vi "test Undeployment Returns to Default State.vi"(8 "error in (no error)":errorcluster, 11 "TestCase in":refnum<class "NI-SWITCH System Tests.lvclass">) -> (0 "error out":errorcluster, 3 "TestCase out":refnum<class "NI-SWITCH System Tests.lvclass">)   [LabVIEW 2017, in "NI-SWITCH System Tests.lvclass"]
uses:
  NI-SWITCH System Tests.lvclass
  SLSC Switch States.ctl
  NI-SWITCH System Tests.lvclass/NI-SWITCH System Tests.ctl
  <vilib>/addons/_JKI Toolkits/VI Tester/TestCase.llb/TestCase.lvclass
  C:/Program Files (x86)/National Instruments/LabVIEW 2017/vi.lib/addons/_JKI Toolkits/VI Tester/TestCase.llb/TestCase.lvclass
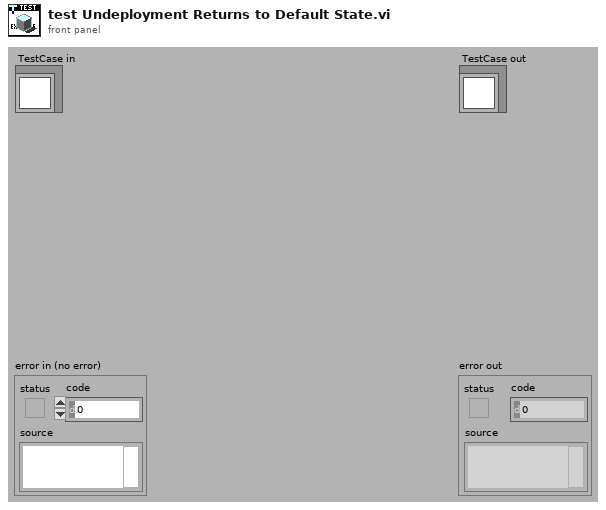
[diagram p1: front panel]
types:
  T1 = typedef "NI-SWITCH System Tests.lvclass/SLSC Switch States.ctl" = cluster{"Channel Load States":cluster{"name":string, "value":i32}[], "Channel Bus States":cluster{"name":string, "value":i32}[], "Channel Pair States":cluster{"name":string, "value":i32}[]}
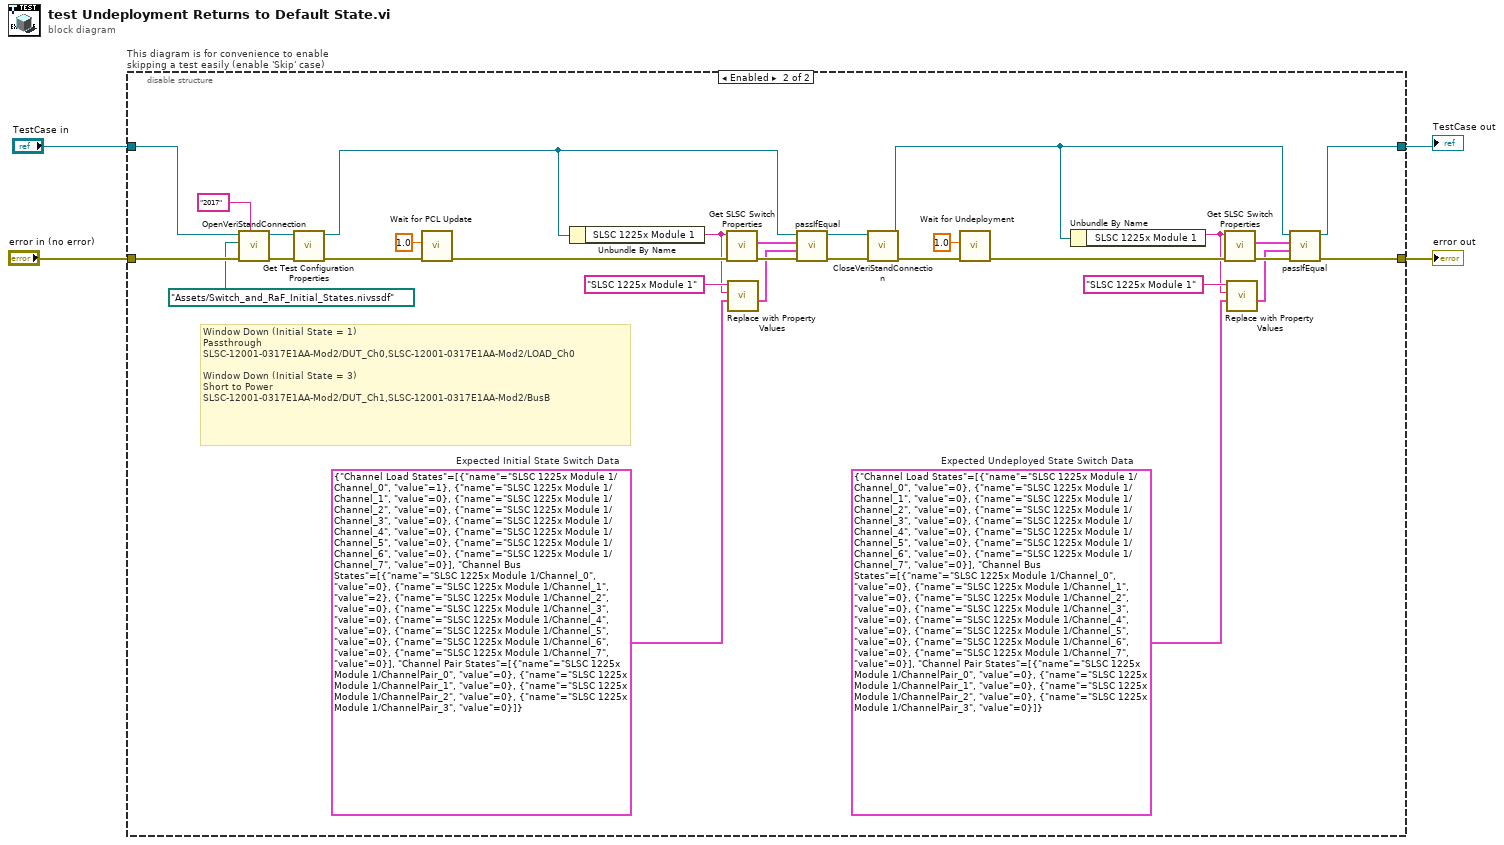
[diagram p0: block diagram]
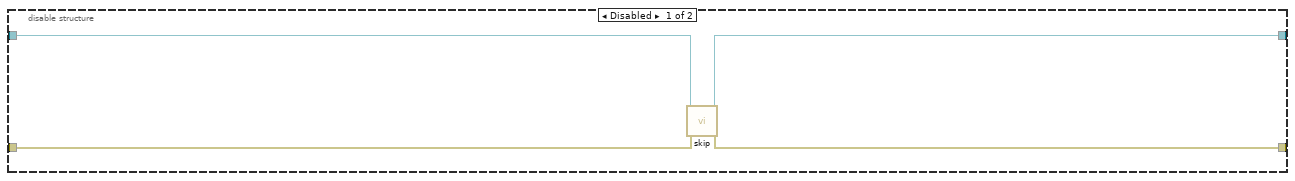
[diagram p2: hidden frame]
diagram:
  n1 = disable-structure "This diagram is for convenience to enable skipping a test easily (enable 'Skip' case)" shown="Enabled" {
    disable-tunnel: "TestCase in" -> [w8 w37]
    disable-tunnel: [w7 w22] -> w2
    disable-tunnel: [w6 w23] -> w1
    disable-tunnel: "error in (no error)" -> [w5 w36]
    frame Disabled {
      n2 = call <vilib>:"skip.vi"("error in (no error)"=w5, "TestCase in"=w8) -> ("error out"=w6:errorcluster, "TestCase out"=w7:refnum<class "NI-SWITCH System Tests.lvclass">)  [unwired: 8 in]
    }
    frame Enabled {
      w11 = T1 {"Channel Load States"=[{"name"="SLSC 1225x Module 1/Channel_0", "value"=0}, {"name"="SLSC 1225x Module 1/Channel_1", "value"=0}, {"name"="SLSC 1225x Module 1/Channel_2", "value"=0}, {"name"="SLSC 1225x Module 1/Channel_3", "value"=0}, {"name"="SLSC 1225x Module 1/Channel_4", "value"=0}, {"name"="SLSC 1225x Module 1/Channel_5", "value"=0}, {"name"="SLSC 1225x Module 1/Channel_6", "value"=0}, {"name"="SLSC 1225x Module 1/Channel_7", "value"=0}], "Channel Bus States"=[{"name"="SLSC 1225x Module 1/Channel_0", "value"=0}, {"name"="SLSC 1225x Module 1/Channel_1", "value"=0}, {"name"="SLSC 1225x Module 1/Channel_2", "value"=0}, {"name"="SLSC 1225x Module 1/Channel_3", "value"=0}, {"name"="SLSC 1225x Module 1/Channel_4", "value"=0}, {"name"="SLSC 1225x Module 1/Channel_5", "value"=0}, {"name"="SLSC 1225x Module 1/Channel_6", "value"=0}, {"name"="SLSC 1225x Module 1/Channel_7", "value"=0}], "Channel Pair States"=[{"name"="SLSC 1225x Module 1/ChannelPair_0", "value"=0}, {"name"="SLSC 1225x Module 1/ChannelPair_1", "value"=0}, {"name"="SLSC 1225x Module 1/ChannelPair_2", "value"=0}, {"name"="SLSC 1225x Module 1/ChannelPair_3", "value"=0}]}  # Expected Undeployed State Switch Data
      w10 = T1 {"Channel Load States"=[{"name"="SLSC 1225x Module 1/Channel_0", "value"=1}, {"name"="SLSC 1225x Module 1/Channel_1", "value"=0}, {"name"="SLSC 1225x Module 1/Channel_2", "value"=0}, {"name"="SLSC 1225x Module 1/Channel_3", "value"=0}, {"name"="SLSC 1225x Module 1/Channel_4", "value"=0}, {"name"="SLSC 1225x Module 1/Channel_5", "value"=0}, {"name"="SLSC 1225x Module 1/Channel_6", "value"=0}, {"name"="SLSC 1225x Module 1/Channel_7", "value"=0}], "Channel Bus States"=[{"name"="SLSC 1225x Module 1/Channel_0", "value"=0}, {"name"="SLSC 1225x Module 1/Channel_1", "value"=2}, {"name"="SLSC 1225x Module 1/Channel_2", "value"=0}, {"name"="SLSC 1225x Module 1/Channel_3", "value"=0}, {"name"="SLSC 1225x Module 1/Channel_4", "value"=0}, {"name"="SLSC 1225x Module 1/Channel_5", "value"=0}, {"name"="SLSC 1225x Module 1/Channel_6", "value"=0}, {"name"="SLSC 1225x Module 1/Channel_7", "value"=0}], "Channel Pair States"=[{"name"="SLSC 1225x Module 1/ChannelPair_0", "value"=0}, {"name"="SLSC 1225x Module 1/ChannelPair_1", "value"=0}, {"name"="SLSC 1225x Module 1/ChannelPair_2", "value"=0}, {"name"="SLSC 1225x Module 1/ChannelPair_3", "value"=0}]}  # Expected Initial State Switch Data
      # "Window Down (Initial State = 1)\nPassthrough\nSLSC-12001-0317E1AA-Mod2/DUT_Ch0,SLSC-12001-0317E1AA-Mod2/LOAD_Ch0\n\nWindow Down (Initial State = 3)\nShort to Power\nSLSC-12001-0317E1AA-Mod2/DUT_Ch1,SLSC-12001-0317E1AA-Mod2/BusB"
      n3 = call-dynamic "OpenVeriStandConnection.vi"("Minimum VeriStand Version (2016)"="2017" ("Minimum VeriStand Version (2015)"), "error in (no error)"=w36, "System Definition File"=path "Assets/Switch_and_RaF_Initial_States.nivssdf", "VeriStand Test Case in"=w37) -> ("error out"=w30:errorcluster, "VeriStand Test Case out"=w19:refnum<class "NI-SWITCH System Tests.lvclass">)  [unwired: 5 in, 1 out]
      n4 = call "Get Test Configuration Properties.vi"("error in (no error)"=w30, "Routing and Faulting System Tests in"=w19) -> ("error out"=w20:errorcluster, "Routing and Faulting System Tests out"=w18:refnum<class "NI-SWITCH System Tests.lvclass">)  [unwired: 8 in]
      n5 = call "Wait for PCL Update"("error in (no error)"=w20, "Delay Time (s)"=1.0) -> ("error out"=w29:errorcluster)  [unwired: 9 in]
      n6 = Unbundle By Name(w18) -> ("SLSC 1225x Module 1"=w9:string)
      n7 = call "Get SLSC Switch Properties.vi"("error in (no error)"=w29, "device"=w9) -> ("error out"=w34:errorcluster, "SLSC Switch States"=w33:T1)  [unwired: 8 in]
      n8 = call "Replace with Property Values.vi"("SLSC Switch States in"=w10, "replace string"=w9, "search string"="SLSC 1225x Module 1" ("name")) -> ("SLSC Switch States out"=w14:T1)  [unwired: 8 in]
      n9 = call-dynamic "passIfEqual.vi"("error in (no error)"=w34, "y"=w14, "x"=w33, "TestCase in"=w18) -> ("error out"=w31:errorcluster, "TestCase out"=w32:refnum<class "NI-SWITCH System Tests.lvclass">)  [unwired: 6 in]
      n10 = call-dynamic "CloseVeriStandConnection.vi"("error in (no error)"=w31, "VeriStand Test Case in"=w32) -> ("error out"=w26:errorcluster, "VeriStand Test Case out"=w17:refnum<class "NI-SWITCH System Tests.lvclass">)  [unwired: 8 in]
      n11 = call "Wait for Undeployment"("error in (no error)"=w26, "Delay Time (s)"=1.0) -> ("error out"=w25:errorcluster)  [unwired: 9 in]
      n12 = Unbundle By Name(w17) -> ("SLSC 1225x Module 1"=w12:string)
      n13 = call "Get SLSC Switch Properties.vi"("error in (no error)"=w25, "device"=w12) -> ("error out"=w24:errorcluster, "SLSC Switch States"=w21:T1)  [unwired: 8 in]
      n14 = call "Replace with Property Values.vi"("SLSC Switch States in"=w11, "replace string"=w12, "search string"="SLSC 1225x Module 1" ("name")) -> ("SLSC Switch States out"=w13:T1)  [unwired: 8 in]
      n15 = call-dynamic "passIfEqual.vi"("error in (no error)"=w24, "y"=w13, "x"=w21, "TestCase in"=w17) -> ("error out"=w23:errorcluster, "TestCase out"=w22:refnum<class "NI-SWITCH System Tests.lvclass">)  [unwired: 6 in]
    }
  }
  "error out" <- w1
  "TestCase out" <- w2
